vi "Stop Actor.vi"(8 "error in":errorcluster) -> (0 "error out":errorcluster)   [LabVIEW 2019, in "ASCII Actor.lvlib"]
uses:
  ASCII Actor.lvlib
  Actor Task.ctl
  Actor Command.ctl
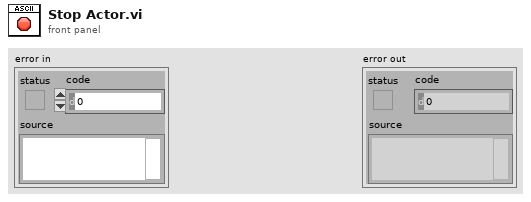
[diagram p1: front panel]
types:
  T1 = typedef "ASCII Actor.lvlib/Actor Task.ctl" = enum8{"Write", "Get Data", "Stop"}
  T2 = typedef "ASCII Actor.lvlib/Actor Command.ctl" = cluster{"Task":T1, "Data":string, "Response Queue":refnum<queue>}
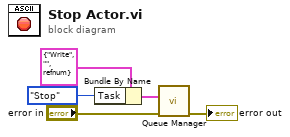
[diagram p0: block diagram]
diagram:
  n1 = Bundle By Name(cluster=T2 {"Task"=enum."Write", "Data"="", "Response Queue"=refnum} ("Command"), "Task"=Actor_Task."Stop") -> (w1:T2)
  n2 = call "Queue Manager.vi"("error in"="error in", "Command"=w1) -> ("error out"=→"error out":errorcluster)  [unwired: 8 in, 1 out]
